vi "demo.vi"() -> ()   [LabVIEW 2020]
uses:
  ZLGCAN/ControlCAN/Device.ctl
  ZLGCAN/ZLGCAN.lvclass
panel:
  in  "等待回复(T)":bool=TRUE
  out "error Out":errorcluster caption="error IO"
  out "消极响应？":bool
  out "Data Out":u8[](array[numeric]) format="%x"
  in  "Extended?":bool=TRUE
  in  "Receive ID":u32=417001744 format="%x"
  in  "Send ID":u32=416944369 format="%x"
  in  "Data In":u8[](array[numeric])=[16, 131] format="%x"
  in  "CAN Device In":T1={"Device Type"=20, "Device Index"=0, "CANInd"=0, "Baud(E_U)"=1835016} {"Baud(E_U)" items=["1000Kbps"=393219, "800Kbps"=393220, "500Kbps"=393223, "250Kbps"=1835016, "125Kbps"=1835025, "100Kbps"=1441827, "50Kbps"=1835052, "20Kbps"=1441971, "10Kbps"=1835232, "5Kbps"=1835457]; "Device Type" items=["PCI5121"=1, "PCI9810"=2, "USBCAN1"=3, "USBCAN2"=4, "PCI9820"=5, "PCI5110"=7, "PC104CAN"=11, "CANETUDP"=12, "PCI9840B"=14, "PC104C2"=15, "PCI9820I"=16, "CANETTCP"=17, "PCIE9221"=24, "PCI5010U"=19, "USBCAN_E_U"=20, "USBCAN_2E_U"=21, "PCI5020U"=22, "PCIE9120I"=27, "PCIE9110I"=28, "PCIE9140I"=29, "USBCAN-4E-U"=31, "USBCAN-8E-U"=34]}
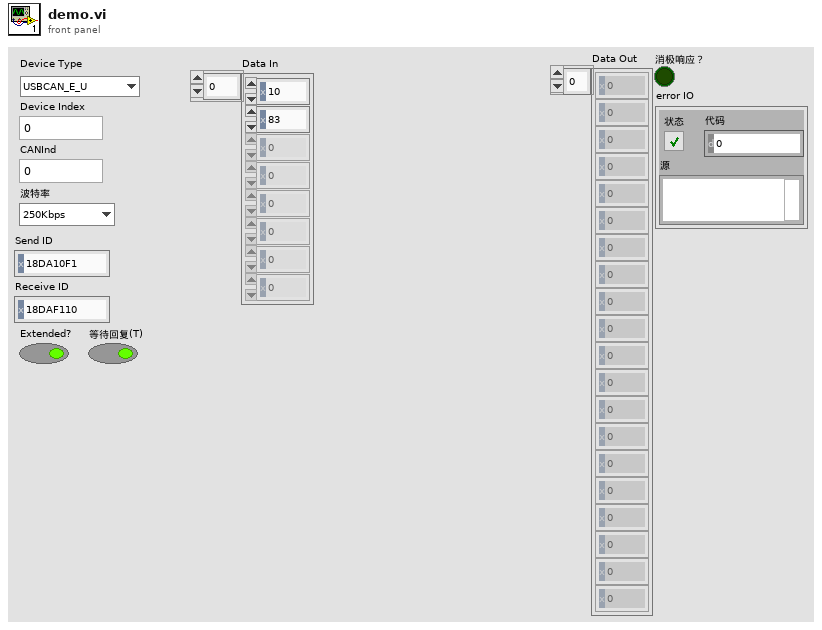
[diagram p1: front panel]
types:
  T1 = typedef "ZLGCAN.lvclass/Device.ctl" = cluster{"Device Type":u32, "Device Index":u32, "CANInd":u32, "Baud(E_U)":u32}
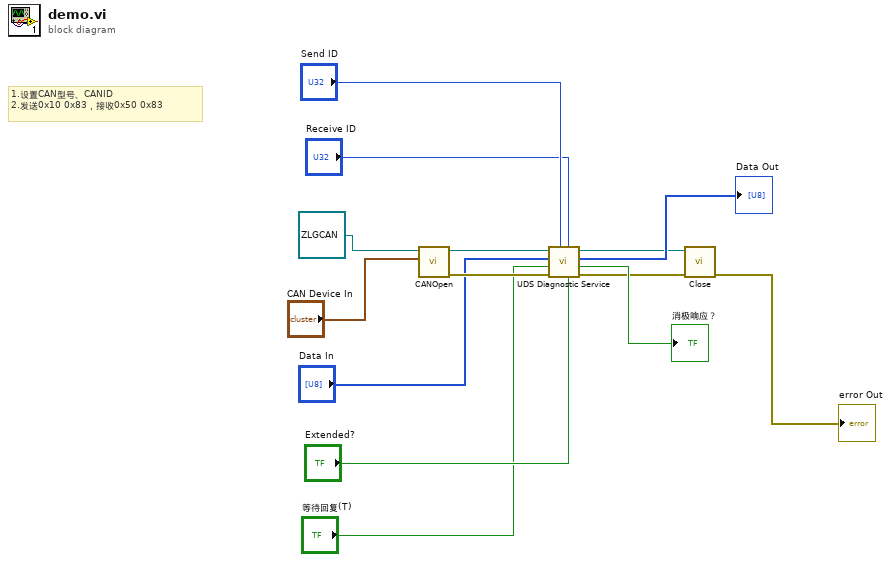
[diagram p0: block diagram]
diagram:
  # "1.设置CAN型号、CANID\n2.发送0x10 0x83，接收0x50 0x83"
  n1 = call "CANOpen.vi"("CAN Device In"="CAN Device In", "ZLGCAN 输入"=refnum<class "ZLGCAN.lvclass"> refnum ("ZLGCAN.lvclass")) -> ("error out"=w12:errorcluster, "ZLGCAN 输出"=w13:refnum<class "ZLGCAN.lvclass">)  [unwired: 8 in]
  n2 = call "UDS Diagnostic Service.vi"("Extended?"="Extended?", "Receive ID"="Receive ID", "Send ID"="Send ID", "Error In"=w12, "等待回复(T)"="等待回复(T)", "Data In"="Data In", "CANIn"=w13) -> ("error Out"=w3:errorcluster, "消极响应？"=→"消极响应？":bool, "Data Out"=→"Data Out":u8[], "CANOut"=w4:refnum<class "ZLGCAN.lvclass">)  [unwired: 1 in]
  n3 = call-dynamic "Close.vi"("error in (no error)"=w3, "ZLGCAN 输入"=w4) -> ("error out"=→"error Out":errorcluster)  [unwired: 8 in, 1 out]
